vi "getTaskRef.vi"(8 "error in (no error)":errorcluster, 11 "niDAQmxAO.lvclass in":refnum<class "niDAQmxAO.lvclass">) -> (0 "error out":errorcluster, 2 "DAQmx Task Ref":refnum<k21>, 3 "niDAQmxAO.lvclass out":refnum<class "niDAQmxAO.lvclass">)   [LabVIEW 2011, in "Hardware.lvlib" / "Channels.lvlib" / "niDAQmxAO.lvclass"]
uses:
  niDAQmxAO.lvclass
  niDAQmxAO.lvclass/niDAQmxAO.ctl
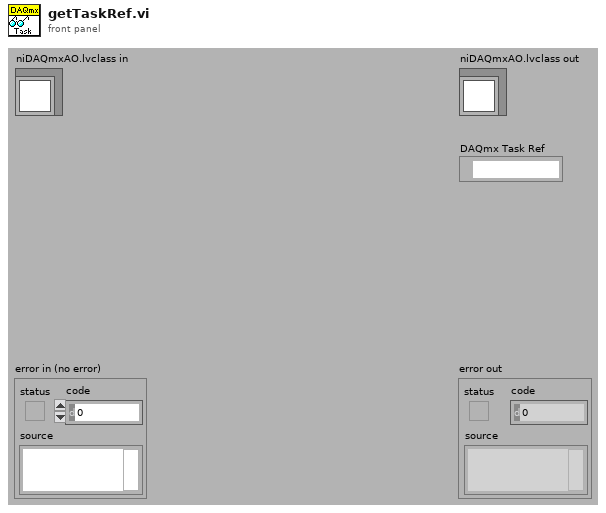
[diagram p1: front panel]
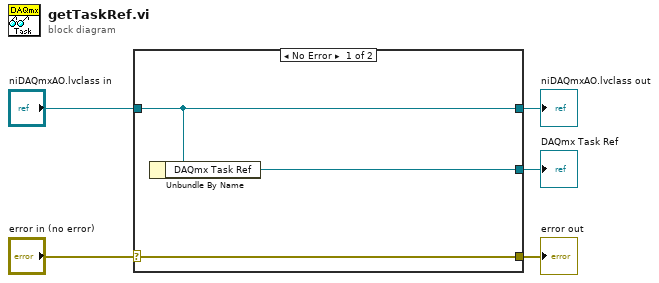
[diagram p0: block diagram]
diagram:
  n1 = case shown="No Error" "error in (no error)" {
    selector: "error in (no error)" -> [w8 w9]
    tunnel: [w8 w9] -> w4
    tunnel: [w7 w10] -> w2
    tunnel: "niDAQmxAO.lvclass in" -> [w7 w10]
    tunnel: [w6 _] -> w1
    frame No Error {
      n2 = Unbundle By Name(w7) -> ("DAQmx Task Ref"=w6:refnum<k21>)
    }
    frame Error {
    }
  }
  "error out" <- w4
  "niDAQmxAO.lvclass out" <- w2
  "DAQmx Task Ref" <- w1
